vi "dvp Vi Get Contrast State.vi"(10 "pContrastState":i32, 11 "handle":u32) -> (2 "pContrastState out":i32, 3 "function return":u32(ring))   [LabVIEW 2018, in "LabViewDVPCamera.lvlib"]
doc: "LabviewDvp2Api dvpStatus dvpViGetContrastState(dvpHandle handle, BOOL *pContrastState);"
uses:
  LabViewDVPCamera.lvlib
  LabViewDVPCamera/LabViewDVPCamera.dll
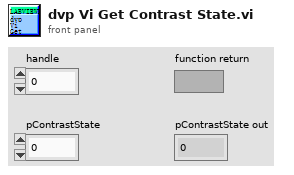
[diagram p1: front panel]
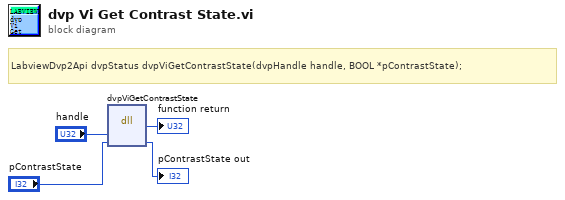
[diagram p0: block diagram]
diagram:
  # "LabviewDvp2Api dvpStatus dvpViGetContrastState(dvpHandle handle, BOOL *pContrastState);"
  n1 = dll-call lib="C:/Program Files (x86)/DVP2 Labview cn 64/Sample/LabViewDVPCamera/LabViewDVPCamera.*" fn="dvpViGetContrastState"("handle"="handle", "pContrastState"="pContrastState") -> (→"function return":u32, "pContrastState"=→"pContrastState out":i32)  [unwired: 4 in, 2 out]
